vi "Teleop.vi"(10 "Match Info":T4={"Autonomous Elapsed Seconds"=0.0, "TeleOp Elapsed Seconds"=0.0, "Disabled Elapsed Seconds"=0.0, "Visited Autonomous"=FALSE, "Visited TeleOp"=FALSE, "Visited Disabled"=FALSE, "Autonomous Settings"={"Autonomous Style"=enum."Independent", "VI Refnum"=refnum}}, 11 "Call Context":T5) -> ()   [LabVIEW 2014]
doc: "This VI is called for each TeleOp packet received from the DS where the robot is not disabled. It is often used to read from the joysticks and update I/O or to update setpoints for timed control loops. It should complete and return within 20 milliseconds or it may miss DS packets."
uses:
  <vilib>/Rock Robotics/WPI/DriverStation/WPI_DriverStationDerivedRobotMode.ctl
  <vilib>/Rock Robotics/WPI/DriverStation/WPI_DriverStationMatch Info.ctl
  Test Typ Def.ctl
  <vilib>/Rock Robotics/Network Tables/SD Read Boolean.vi
  <vilib>/Rock Robotics/Network Tables/SD Read Number.vi
  <vilib>/Rock Robotics/WPI/Joystick/WPI_JoystickGetSetRefNum.vi
  <vilib>/Rock Robotics/Network Tables/SD Write Boolean.vi
  <vilib>/Rock Robotics/Network Tables/SD Write Numeric Array.vi
panel:
  out "Axes Indicator":T1
  out "Manipulator State 2":T2(ring)
  in  "Claw Opened Limit":bool
  in  "Claw Closed Limit":bool
  in  "Bottom Limit":bool
  in  "Top Limit":bool
  in  "Button b":bool
  in  "Button a":bool
  in  "point reached":bool
  out "Time For Manipulator":dbl
  in  "Button y":bool
  in  "Button x":bool
  in  "Manipulator State":T3
  out "error out 2":errorcluster
  out "current (A)":dbl
  out "all currents (A)":dbl[](array[numeric])
  out "Power (W)":dbl
  out "error out 5":errorcluster
  out "Buttons":bool[](array[boolean])
  out "Sample Slider 0":dbl(slide) scale=0.0..5.0
  out "Sample Boolean 1":bool
  out "Sample Boolean 0":bool
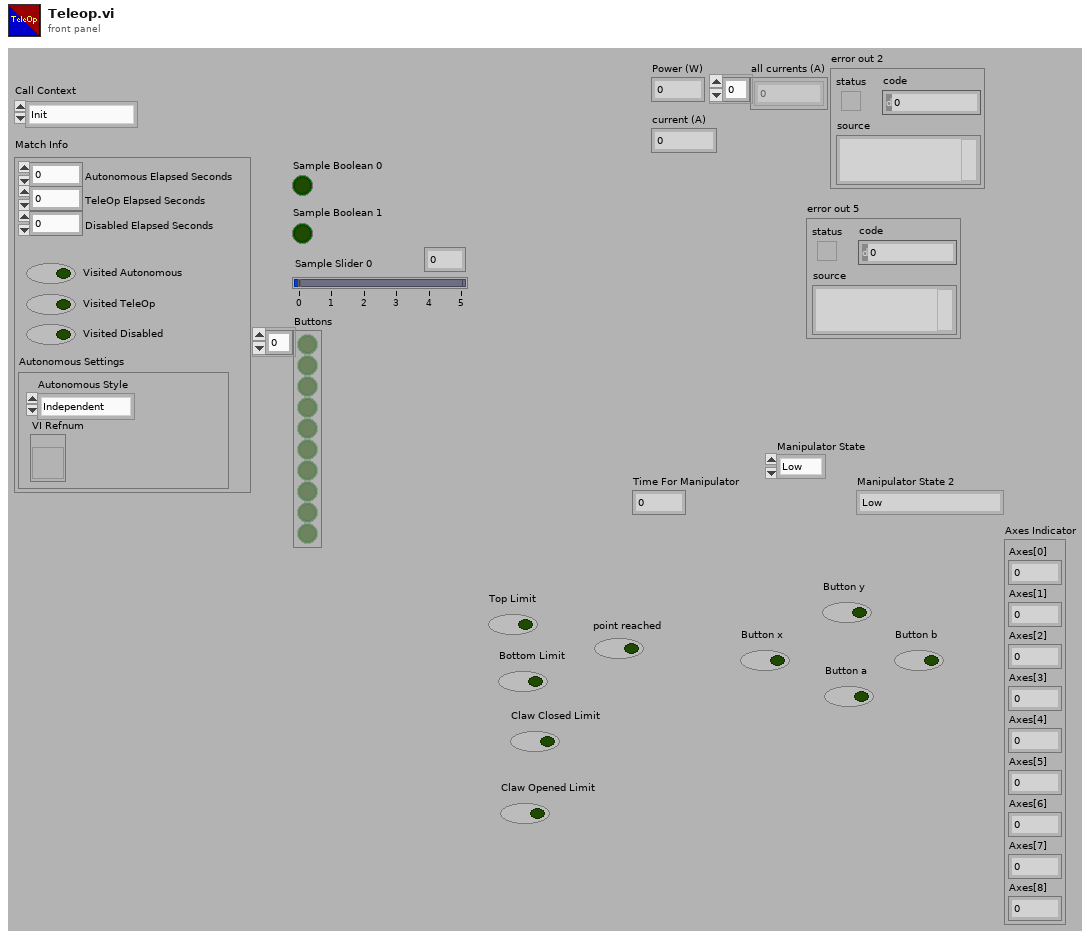
[diagram p1: front panel]
types:
  T1 = cluster{"Axes[0]":dbl, "Axes[1]":dbl, "Axes[2]":dbl, "Axes[3]":dbl, "Axes[4]":dbl, "Axes[5]":dbl, "Axes[6]":dbl, "Axes[7]":dbl, "Axes[8]":dbl}
  T2 = enum16{"Low", "RC Close", "Tote Close", "RC High", "Tote High", "Lowering", "Opening", "RC Top Stacker", "Bottom Stacking", "RC raising", "Tote Raising", "Limit High"}
  T3 = typedef "Test Typ Def.ctl" = enum16{"Low", "RC Close", "Tote Close", "RC High", "Tote High", "Lowering", "Opening", "RC Top Stacker", "Bottom Stacking", "RC raising", "Tote Raising", "Limit High"}
  T4 = typedef "WPI_DriverStationMatch Info.ctl" = cluster{"Autonomous Elapsed Seconds":dbl, "TeleOp Elapsed Seconds":dbl, "Disabled Elapsed Seconds":dbl, "Visited Autonomous":bool, "Visited TeleOp":bool, "Visited Disabled":bool, "Autonomous Settings":cluster{"Autonomous Style":enum16{"Iterative", "Independent"}, "VI Refnum":refnum<vi>}}
  T5 = typedef "WPI_DriverStationDerivedRobotMode.ctl" = enum16{"Init", "Execute", "Stop"}
  T6 = typedef "WPI_JoystickDevRef.ctl" = cluster{"Device":T7}
  T7 = typedef "WPI_JoystickDeviceEnum.ctl" = enum16{"USB 0", "USB 1", "USB 2", "USB 3", "USB 4", "USB 5"}
  T8 = enum16{"Low", "RC Close", "Tote Close", "RC High", "Tote High", "Lowering", "Opening", "RC Top Stacker", "Bottom Stacking"}
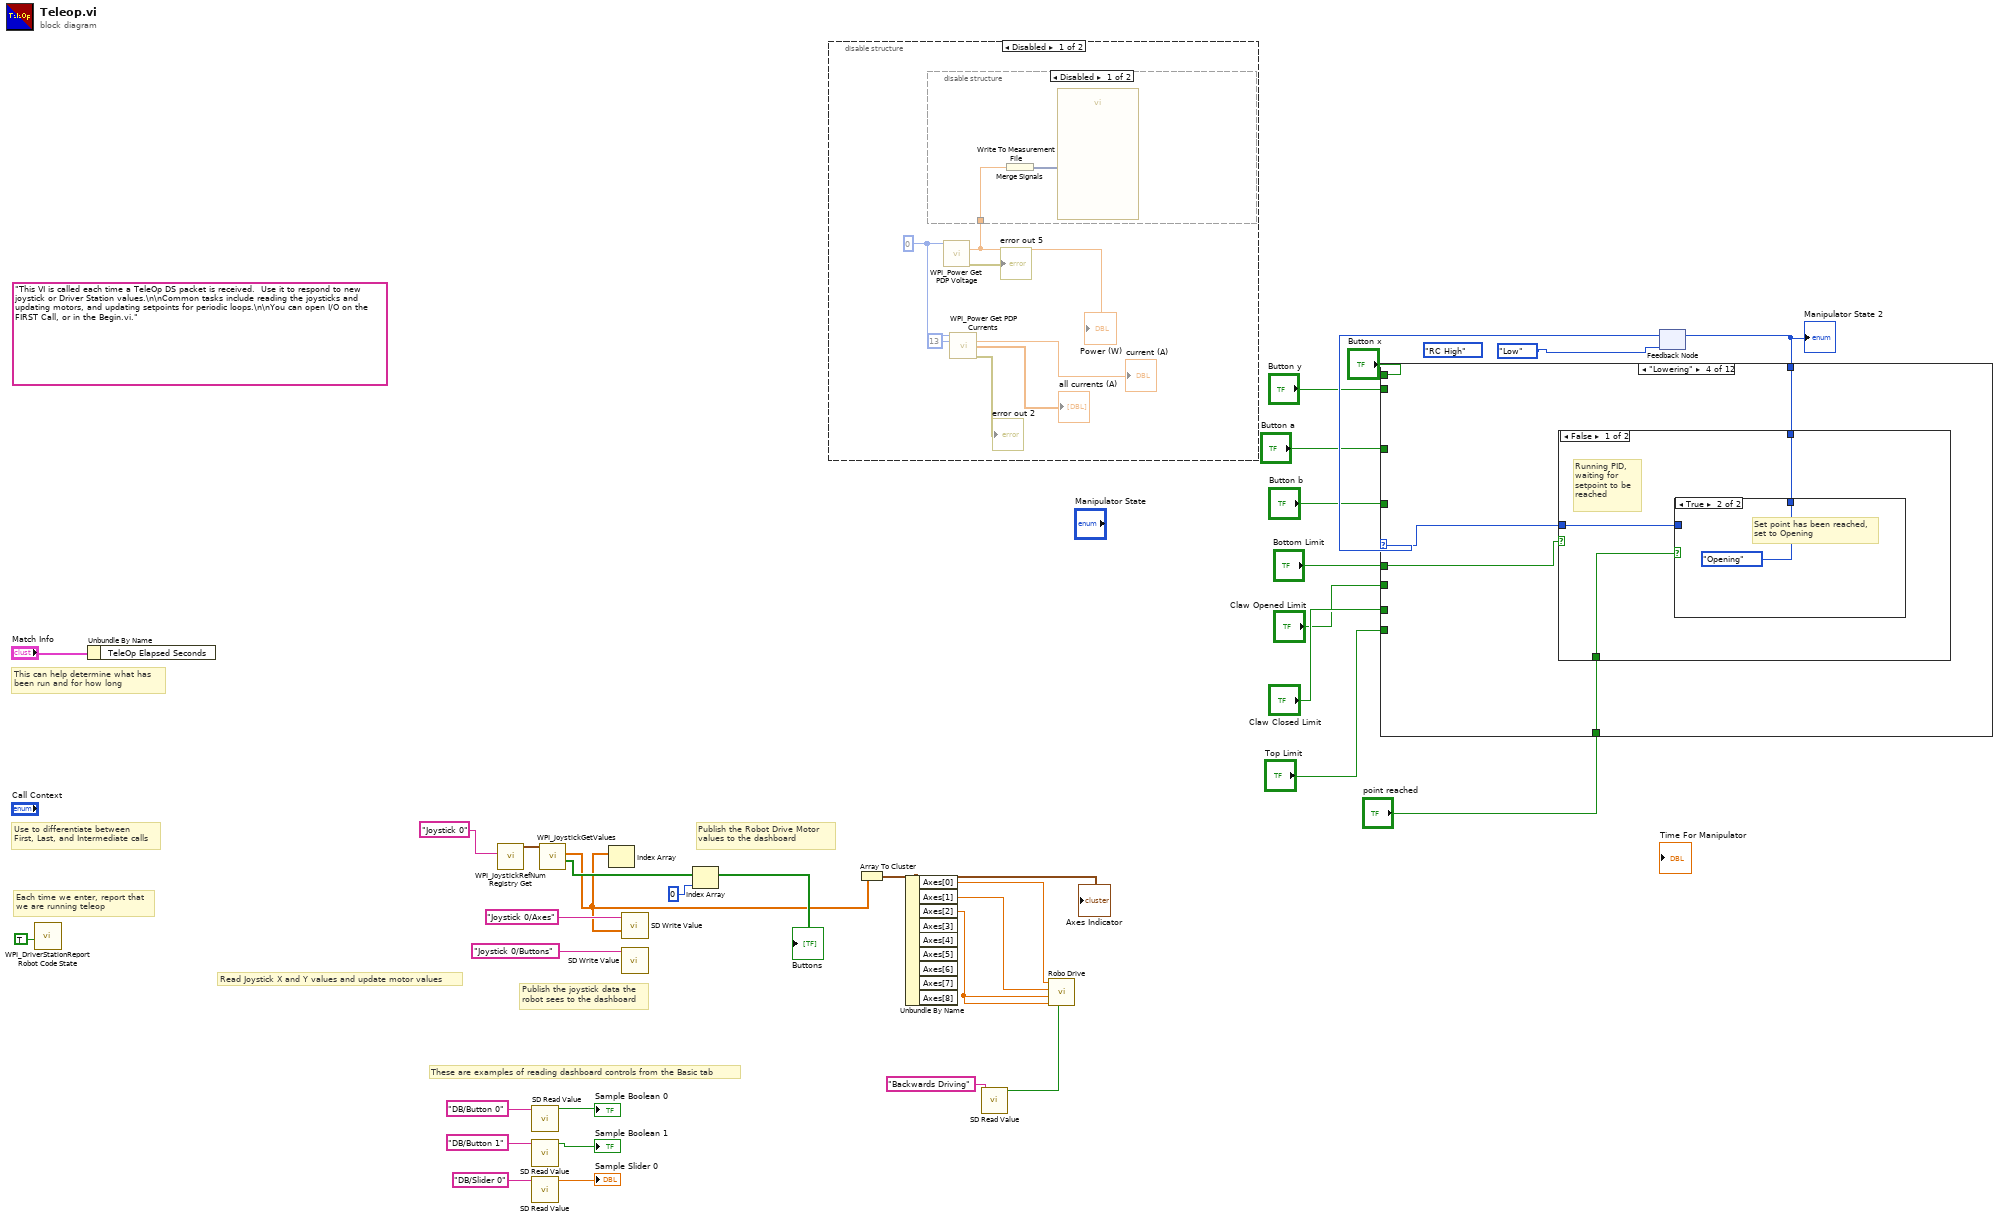
[diagram p0: block diagram]
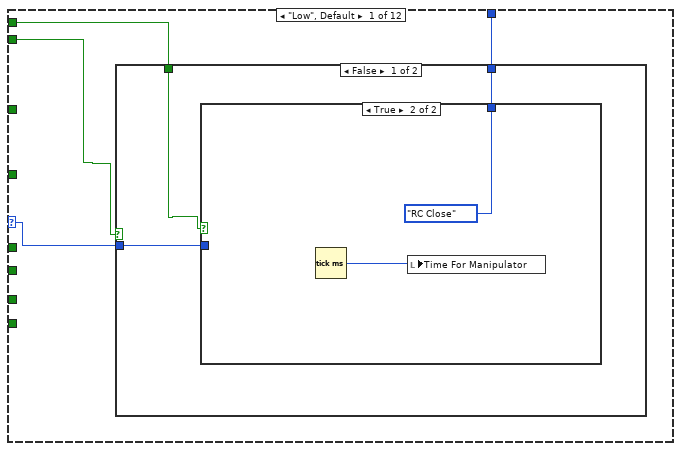
[diagram p2: hidden frame]
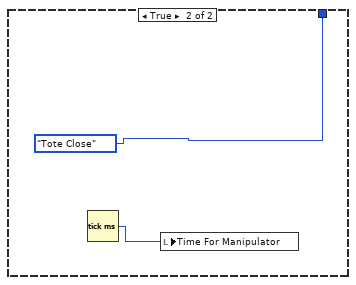
[diagram p4: hidden frame]
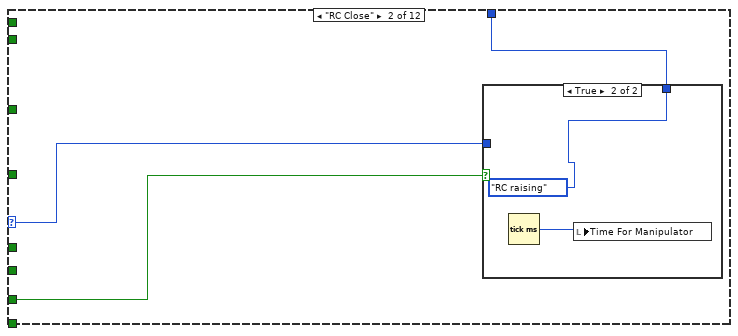
[diagram p5: hidden frame]
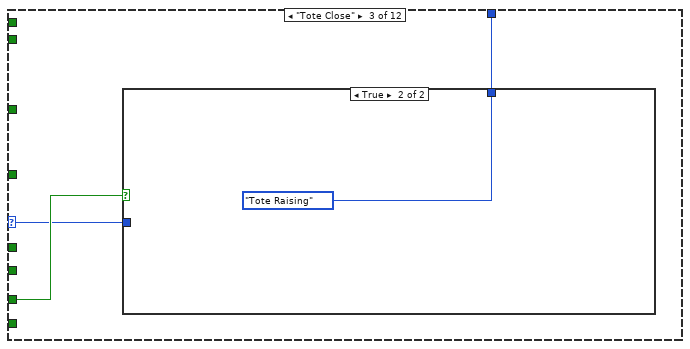
[diagram p7: hidden frame]
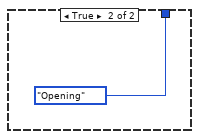
[diagram p10: hidden frame]
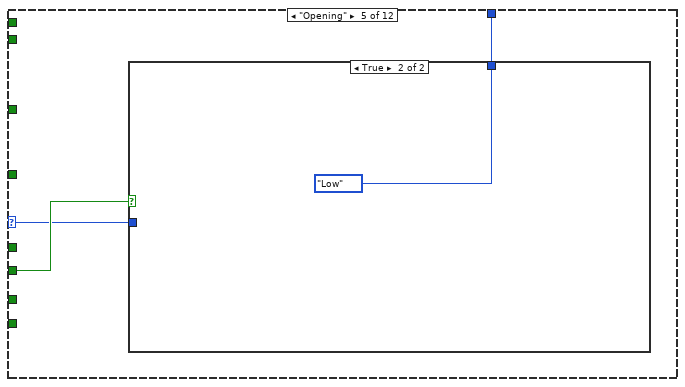
[diagram p11: hidden frame]
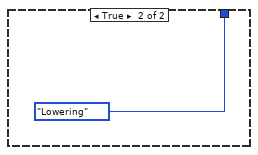
[diagram p14: hidden frame]
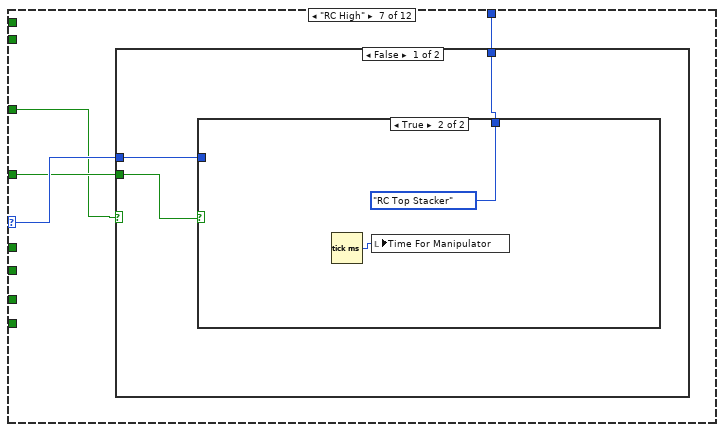
[diagram p15: hidden frame]
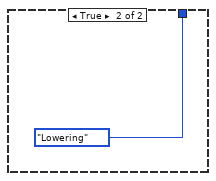
[diagram p17: hidden frame]
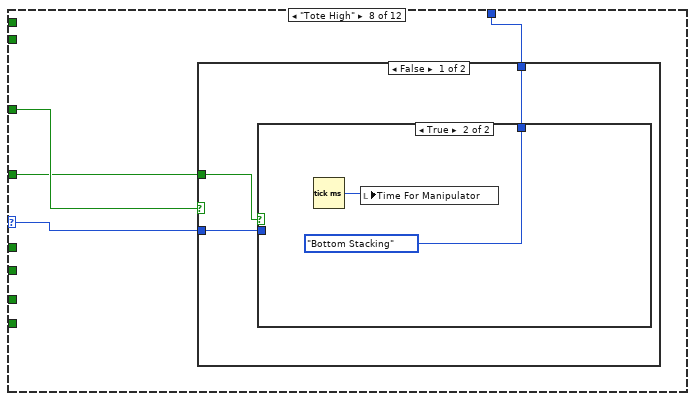
[diagram p18: hidden frame]
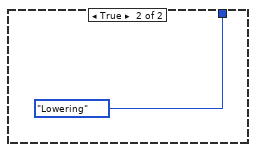
[diagram p20: hidden frame]
diagram:
  (unwired) Test_Typ_Def."RC High" ("Manipulator State")
  (unwired) "This VI is called each time a TeleOp DS packet is received.  Use it to respond to new joystick or Driver Station values.\n\nCommon tasks include reading the joysticks and updating motors, and updating setpoints for periodic loops.\n\nYou can open I/O on the FIRST Call, or in the Begin.vi."
  # "Publish the Robot Drive Motor\nvalues to the dashboard"
  # "Publish the joystick data the\nrobot sees to the dashboard"
  # "Read Joystick X and Y values and update motor values"
  # "These are examples of reading dashboard controls from the Basic tab"
  # "Each time we enter, report that\nwe are running teleop"
  # "Use to differentiate between\nFirst, Last, and Intermediate calls"
  # "This can help determine what has\nbeen run and for how long"
  n1 = call <vilib>:"WPI_DriverStationReport Robot Code State.vi"("TeleOp"=TRUE ("Autonomous")) -> ()  [unwired: 10 in, 1 out]
  n2 = Unbundle By Name("Match Info") -> ()  [unwired: 1 out]
  n3 = call <vilib>:"WPI_JoystickRefNum Registry Get.vi"("refnum name"="Joystick 0") -> ("JoystickDevRef"=w13:T6)  [unwired: 1 in, 9 out]
  n4 = call-poly <vilib>:"SD Read Value.vi"("Name"="DB/Button 0" ("refnum name")) -> ("Boolean"=→"Sample Boolean 0":bool)  [unwired: 8 in, 2 out]
  n5 = call-poly <vilib>:"SD Read Value.vi"("Name"="DB/Button 1" ("refnum name")) -> ("Boolean"=→"Sample Boolean 1":bool)  [unwired: 8 in, 2 out]
  n6 = call-poly <vilib>:"SD Read Value.vi"("Name"="DB/Slider 0" ("refnum name")) -> ("Numeric"=→"Sample Slider 0":dbl)  [unwired: 8 in, 2 out]
  n7 = call <vilib>:"WPI_JoystickGetValues.vi"("JoystickDevRef"=w13) -> ("Buttons"=w10:bool[], "Axes"=w7:dbl[])  [unwired: 6 in, 3 out]
  "Buttons" <- w10
  n8 = Index Array(array=w7) -> ()  [unwired: 1 in, 1 out]
  n9 = call-poly <vilib>:"SD Write Value.vi"("Numeric Array"=w7, "Name"="Joystick 0/Axes") -> ()  [unwired: 8 in, 2 out]
  n10 = call-poly <vilib>:"SD Write Value.vi"("Name"="Joystick 0/Buttons") -> ()  [unwired: 9 in, 2 out]
  n11 = Index Array(array=w10, index=0) -> ()  [unwired: 1 out]
  n12 = disable-structure shown="Disabled" {
    frame Disabled {
      w38 = u8 0 ("Power Distribution Panel (0)")
      n13 = call <vilib>:"WPI_Power Get PDP Voltage.vi"("Power Distribution Panel (0)"=w38) -> ("voltage (V)"=w40:dbl, "error out"=→"error out 5":errorcluster)  [unwired: 13 in]
      "Power (W)" <- w40
      n14 = disable-structure shown="Disabled" {
        disable-tunnel: w40 -> [w42 _]
        frame Disabled {
          n15 = Merge Signals(w42) -> (w41:dynamicdata)
          n16 = call "Write To Measurement File"("Signals"=w41) -> ()  [unwired: 16 in, 3 out]
        }
        frame Enabled {
        }
      }
      n17 = call <vilib>:"WPI_Power Get PDP Currents.vi"("Power Distribution Panel (0)"=w38, "PDP Channel"=13) -> ("current (A)"=→"current (A)":dbl, "all currents (A)"=→"all currents (A)":dbl[], "error out"=→"error out 2":errorcluster)  [unwired: 11 in]
    }
    frame Enabled {
    }
  }
  n18 = Array To Cluster(array=w7) -> (cluster=w6:T1)
  "Axes Indicator" <- w6
  n19 = Unbundle By Name(w6) -> ("Axes[0]"=w3:dbl, "Axes[1]"=w2:dbl, "Axes[2]"=w1:dbl)  [unwired: 6 out]
  n20 = call-poly <vilib>:"SD Read Value.vi"("Name"="Backwards Driving") -> ("Boolean"=w4:bool)  [unwired: 8 in, 2 out]
  n21 = call "Robo Drive.vi"("Button Flip Directions"=w4, "Right Analog (axes 3)"=w1, "Left Analog (axes 2)"=w1, "Axes 1 (y axis)"=w2, "Axes 0 (x axis)"=w3) -> ()  [unwired: 7 in]
  n22 = feedback #1(T2."Low" ("Manipulator State")) -> (w25:T2)
  n23 = case shown="\"Lowering\"" w25 {
    selector: w25 -> [w43 w56 w61 w66 w76 w81 w89 w99 w108 w117 w128 w136]
    tunnel: [w46 w57 w62 w68 w77 w82 w88 w100 w109 w119 w129 w137] -> w24
    tunnel: "Top Limit" -> [_ _ _ _ _ _ _ _ _ _ w127 w139]
    tunnel: "Bottom Limit" -> [_ _ _ w69 _ _ _ _ _ _ _ _]
    tunnel: "point reached" -> [_ _ _ w67 _ _ _ _ _ _ w126 w138]
    tunnel: "Button b" -> [_ _ _ _ _ _ w87 w97 _ _ _ _]
    tunnel: "Button a" -> [_ _ _ _ _ w83 w86 w98 _ _ _ _]
    tunnel: "Button y" -> [w45 _ _ _ _ _ _ _ _ _ _ _]
    tunnel: "Button x" -> [w44 _ _ _ _ _ _ _ _ _ _ _]
    tunnel: "Claw Closed Limit" -> [_ w55 w63 _ _ _ _ _ _ _ _ _]
    tunnel: "Claw Opened Limit" -> [_ _ _ _ w78 _ _ _ _ _ _ _]
    frame "Low", Default {
      n24 = case shown="False" w45 {
        tunnel: [w49 T2."Tote Close" ("Manipulator State")] -> w46
        tunnel: w44 -> [w48 _]
        tunnel: w43 -> [w47 _]
        frame False {
          n25 = case shown="True" w48 {
            tunnel: [w50 T8."RC Close" ("Manipulator State")] -> w49
            tunnel: w47 -> [w50 _]
            frame False {
            }
            frame True {
              n26 = Tick Count (ms)() -> (millisecond timer value=w51:u32)
              n27 = local write "Time For Manipulator"(w51) -> ()
            }
          }
        }
        frame True {
          n28 = Tick Count (ms)() -> (millisecond timer value=w54:u32)
          n29 = local write "Time For Manipulator"(w54) -> ()
        }
      }
    }
    frame "RC Close" {
      n30 = case shown="True" w55 {
        tunnel: [w58 T2."RC raising" ("Manipulator State")] -> w57
        tunnel: w56 -> [w58 _]
        frame False {
        }
        frame True {
          n31 = Tick Count (ms)() -> (millisecond timer value=w60:u32)
          n32 = local write "Time For Manipulator"(w60) -> ()
        }
      }
    }
    frame "Tote Close" {
      n33 = case shown="True" w63 {
        tunnel: [w64 T2."Tote Raising" ("Manipulator State")] -> w62
        tunnel: w61 -> [w64 _]
        frame False {
        }
        frame True {
        }
      }
    }
    frame "Lowering" {
      n34 = case shown="False" w69 {
        tunnel: [w71 T2."Opening" ("Manipulator State")] -> w68
        tunnel: w67 -> [w72 _]
        tunnel: w66 -> [w70 _]
        frame False {
          # "Running PID,\nwaiting for \nsetpoint to be \nreached"
          n35 = case shown="True" w72 {
            tunnel: [w73 T2."Opening" ("Manipulator State")] -> w71
            tunnel: w70 -> [w73 _]
            frame False {
            }
            frame True {
              # "Set point has been reached,\nset to Opening"
            }
          }
        }
        frame True {
        }
      }
    }
    frame "Opening" {
      n36 = case shown="True" w78 {
        tunnel: [w79 T2."Low" ("Manipulator State")] -> w77
        tunnel: w76 -> [w79 _]
        frame False {
          # "Set Claw Motor To open at half speed"
        }
        frame True {
        }
      }
    }
    frame "Limit High" {
      n37 = case shown="False" w83 {
        tunnel: [w84 T2."Lowering" ("Manipulator State")] -> w82
        tunnel: w81 -> [w84 _]
        frame False {
        }
        frame True {
        }
      }
    }
    frame "RC High" {
      n38 = case shown="False" w86 {
        tunnel: w89 -> [w92 _]
        tunnel: [w91 T2."Lowering" ("Manipulator State")] -> w88
        tunnel: w87 -> [w90 _]
        frame False {
          n39 = case shown="True" w90 {
            tunnel: [w93 T2."RC Top Stacker" ("Manipulator State")] -> w91
            tunnel: w92 -> [w93 _]
            frame False {
            }
            frame True {
              n40 = Tick Count (ms)() -> (millisecond timer value=w94:u32)
              n41 = local write "Time For Manipulator"(w94) -> ()
            }
          }
        }
        frame True {
        }
      }
    }
    frame "Tote High" {
      n42 = case shown="False" w98 {
        tunnel: [w103 T2."Lowering" ("Manipulator State")] -> w100
        tunnel: w99 -> [w102 _]
        tunnel: w97 -> [w101 _]
        frame False {
          n43 = case shown="True" w101 {
            tunnel: [w104 T2."Bottom Stacking" ("Manipulator State")] -> w103
            tunnel: w102 -> [w104 _]
            frame False {
            }
            frame True {
              n44 = Tick Count (ms)() -> (millisecond timer value=w105:u32)
              n45 = local write "Time For Manipulator"(w105) -> ()
            }
          }
        }
        frame True {
        }
      }
    }
    frame "RC Top Stacker" {
      # "This may also include \nbacking up from the completed stack"
      # "Placing RC bin on top of stack, \n1500 ms delay symbolizes this\nfor the sake of this theoretical\nprogram"
      n46 = local read "Time For Manipulator"() -> (w113:dbl)
      n47 = Tick Count (ms)() -> (millisecond timer value=w111:u32)
      n48 = Add(x=1500.0, y=w113) -> (x+y=w112:dbl)
      n49 = Less Or Equal?(x=w112, y=w111) -> (x <= y?=w110:bool)
      n50 = case shown="True" w110 {
        tunnel: [w115 T2."Lowering" ("Manipulator State")] -> w109
        tunnel: w108 -> [w115 _]
        frame False {
        }
        frame True {
        }
      }
    }
    frame "Bottom Stacking" {
      # "This may also include \nbacking up from the completed stack"
      # "Placing RC bin on top of stack, \n1500 ms delay symbolizes this\nfor the sake of this theoretical\nprogram"
      n51 = local read "Time For Manipulator"() -> (w118:dbl)
      n52 = Tick Count (ms)() -> (millisecond timer value=w121:u32)
      n53 = Add(x=1500.0, y=w118) -> (x+y=w122:dbl)
      n54 = Less Or Equal?(x=w122, y=w121) -> (x <= y?=w120:bool)
      n55 = case shown="True" w120 {
        tunnel: [w124 T2."Lowering" ("Manipulator State")] -> w119
        tunnel: w117 -> [w124 _]
        frame False {
        }
        frame True {
        }
      }
    }
    frame "RC raising" {
      n56 = case shown="False" w127 {
        tunnel: [w132 T2."Limit High" ("Manipulator State")] -> w129
        tunnel: w128 -> [w131 _]
        tunnel: w126 -> [w130 _]
        frame False {
          # "Set Point of Manipulator PID\nto height of 'RC high', point\nreached is true when set point \nis reached."
          n57 = case shown="True" w130 {
            tunnel: [w133 T2."RC High" ("Manipulator State")] -> w132
            tunnel: w131 -> [w133 _]
            frame False {
            }
            frame True {
            }
          }
        }
        frame True {
        }
      }
    }
    frame "Tote Raising" {
      n58 = case shown="False" w139 {
        tunnel: w138 -> [w142 _]
        tunnel: [w141 T2."Limit High" ("Manipulator State")] -> w137
        tunnel: w136 -> [w140 _]
        frame False {
          n59 = case shown="True" w142 {
            tunnel: [w143 T2."Tote High" ("Manipulator State")] -> w141
            tunnel: w140 -> [w143 _]
            frame False {
            }
            frame True {
            }
          }
        }
        frame True {
        }
      }
    }
  }
  "Manipulator State 2" <- w24
  n60 = feedback-in #1(w24) -> ()
